vi "Report Start Timing.vi"(5 "VolatusAPI":refnum<class "VolatusAPI.lvclass">, 9 "Seq Name":string, 10 "State Loop Data In":T1, 11 "State in":refnum<class "State.lvclass">) -> (2 "State Loop Data":T1)   [LabVIEW 2023, in "VolatusSeq.lvlib" / "State.lvclass"]
uses:
  State.lvclass
  State.lvclass/State.ctl
  Volatus/VolatusAPI/VolatusAPI.lvclass
  VolatusSeqConfig/Command Type.ctl
  VolatusSeqConfig/VolatusSeqConfig.lvlib
  Volatus/MessageQ/MessageQ.lvclass
  messages/CmdDigital/Data.ctl
  messages/CmdDigital/CmdDigital.lvlib
  messages/CmdAnalog/Data.ctl
  messages/CmdAnalog/CmdAnalog.lvlib
  Send Type.ctl
  VolatusSeq.lvlib
  Command.ctl
  Transition/Transition.lvclass
  Sequence Time.ctl
  Iteration Actions/Iteration Actions.lvclass
  Variables/Variables.lvclass
  State Loop Data.ctl
  lv-vecto/Vecto/Channel DBL/Channel DBL.lvclass
  Format String/Format String.lvclass
  VolatusSeqConfig/Debug Flags.ctl
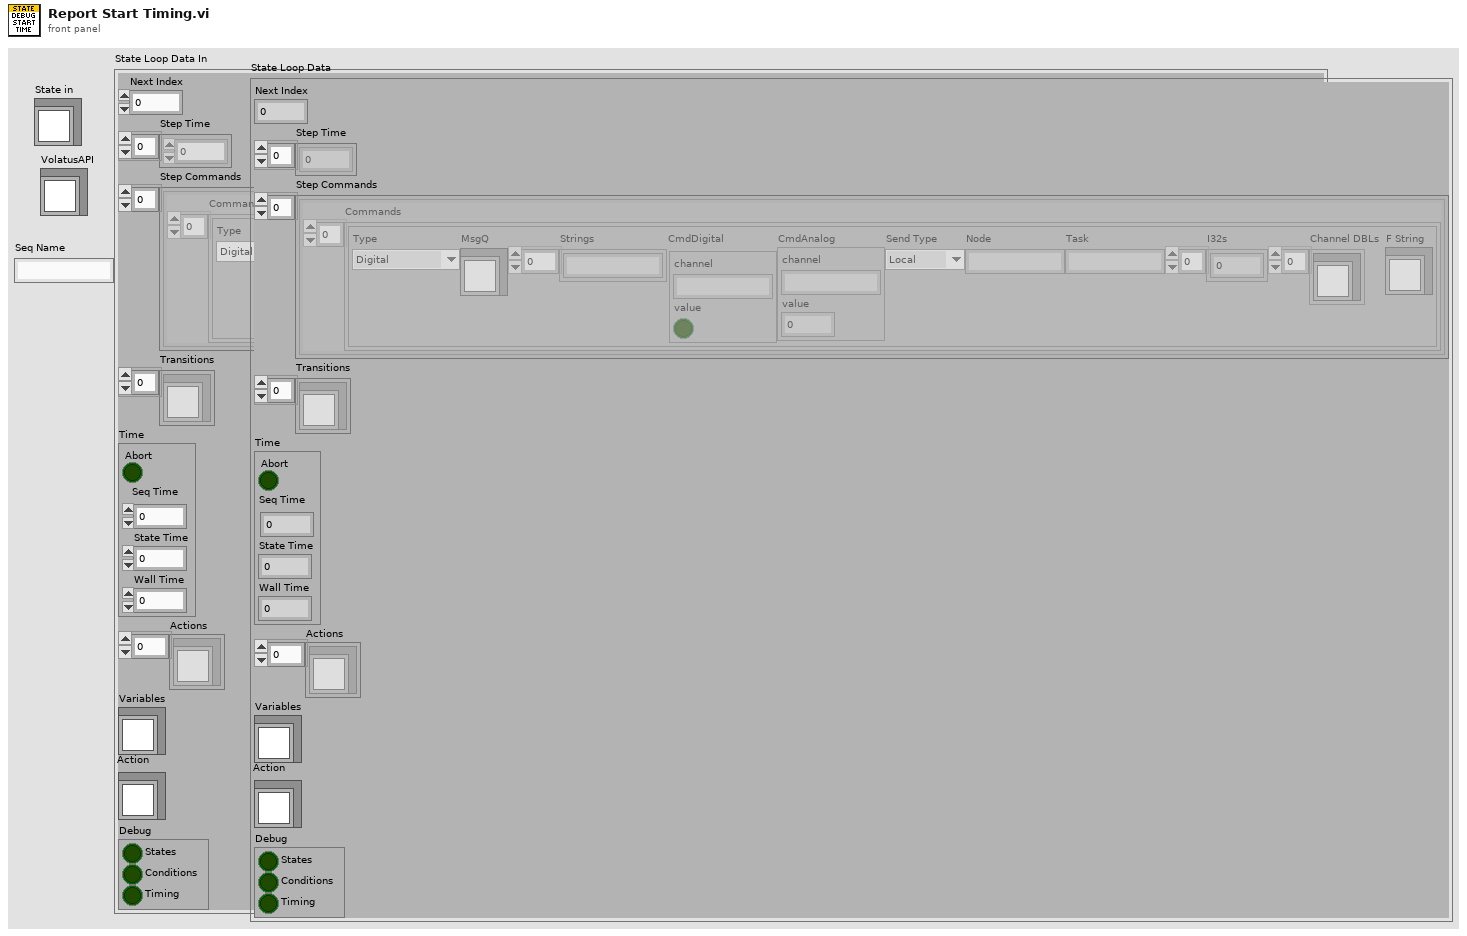
[diagram p1: front panel]
types:
  T1 = typedef "VolatusSeq.lvlib/State.lvclass/State Loop Data.ctl" = cluster{"Next Index":i32, "Step Time":dbl[], "Step Commands":cluster{"Commands":T2[]}[], "Transitions":refnum<class "Transition.lvclass">[], "Time":T7, "Actions":refnum<class "Iteration Actions.lvclass">[], "Variables":refnum<class "Variables.lvclass">, "Action":refnum<class "Iteration Actions.lvclass">, "Debug":T8}
  T2 = typedef "VolatusSeq.lvlib/Command.ctl" = cluster{"Type":T3, "MsgQ":refnum<class "MessageQ.lvclass">, "Strings":string[], "CmdDigital":T4, "CmdAnalog":T5, "Send Type":T6, "Node":string, "Task":string, "I32s":i32[], "Channel DBLs":refnum<class "Channel DBL.lvclass">[], "F String":refnum<class "Format String.lvclass">}
  T3 = typedef "VolatusSeqConfig.lvlib/Command Type.ctl" = enum16{"Digital", "Numeric", "Transition", "Stop", "StartLog", "StopLog", "Start", "Event", "Error", "HTTP", "ResetVar", "IncVar", "DecVar", "SaveVar", "LoadVar", "AddVar", "SubVar", "SetVar", "AddToVar"}
  T4 = typedef "CmdDigital.lvlib/Data.ctl" = cluster{"channel":string, "value":bool}
  T5 = typedef "CmdAnalog.lvlib/Data.ctl" = cluster{"channel":string, "value":dbl}
  T6 = typedef "VolatusSeq.lvlib/Send Type.ctl" = enum16{"Local", "Remote"}
  T7 = typedef "VolatusSeq.lvlib/Sequence Time.ctl" = cluster{"Abort":bool, "Seq Time":dbl, "State Time":dbl, "Wall Time":dbl}
  T8 = typedef "VolatusSeqConfig.lvlib/Debug Flags.ctl" = cluster{"States":bool, "Conditions":bool, "Timing":bool}
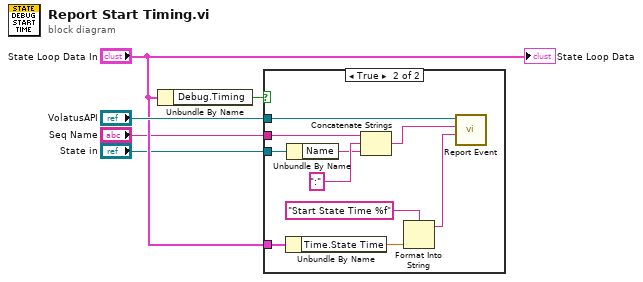
[diagram p0: block diagram]
diagram:
  n1 = Unbundle By Name("State Loop Data In") -> ("Debug.Timing"=w4:bool)
  n2 = case shown="True" w4 {
    tunnel: "VolatusAPI" -> [_ w15]
    tunnel: "State Loop Data In" -> [_ w14]
    tunnel: "Seq Name" -> [_ w12]
    tunnel: "State in" -> [_ w13]
    frame False {
    }
    frame True {
      n3 = Unbundle By Name(w14) -> ("Time.State Time"=w7:dbl)
      n4 = Unbundle By Name(w13) -> ("Name"=w10:string)
      n5 = Concatenate Strings(w12, ":" ("string"), w10) -> (w9:string)
      n6 = Format Into String(format string="Start State Time %f", w7) -> (resulting string=w6:string)  [unwired: 2 in, 1 out]
      n7 = call "Report Event.vi"("Message"=w6, "Context"=w9, "VolatusAPI in"=w15) -> ()  [unwired: 7 in, 2 out]
    }
  }
  "State Loop Data" <- "State Loop Data In"
